vi "MPExxx_Rsrc_example.vi"() -> (0 "Resource String Output":string)   [LabVIEW 2012]
doc: "This VI form creates the resource string for the different communication interfaces."
panel:
  in  "?":T1(tab)
  in  "Comm Port":u8=1 min=1 max=9 step=1
  in  "Address":u8=2 min=1 max=31 step=1
  in  "GPIB Controller":u8
  in  "Port":u16=4000
  in  "TCP/IP Address":string
  # "MAGNA-POWER"
  # "Electronics"
  # "Creates the resource string for ViOpen."
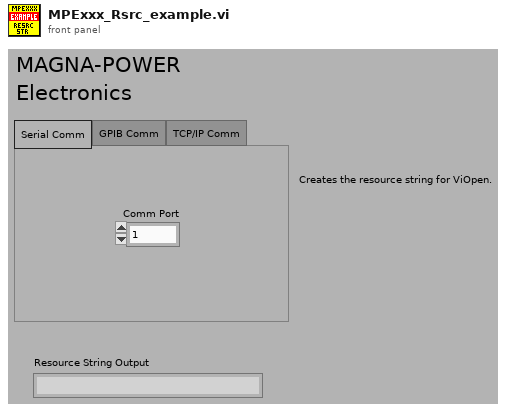
[diagram p1: front panel]
types:
  T1 = enum32{"Serial Comm", "GPIB Comm", "TCP/IP Comm"}
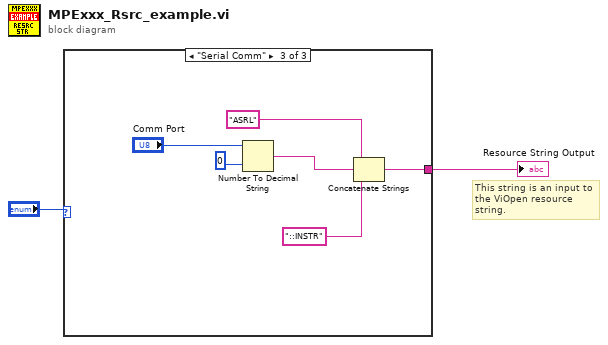
[diagram p0: block diagram]
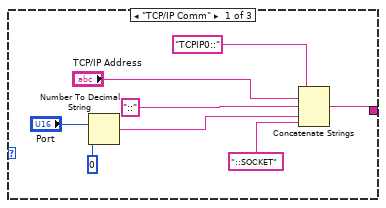
[diagram p2: hidden frame]
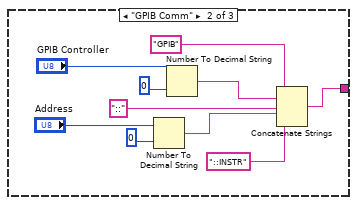
[diagram p3: hidden frame]
diagram:
  # "This string is an input to the ViOpen resource string."
  n1 = case "Case" shown="\"Serial Comm\"" "?" {
    tunnel: [w3 w19 w23] -> w1
    frame "TCP/IP Comm" {
      n2 = Number To Decimal String(number="Port", width (-)=0) -> (decimal integer string=w5:string)
      n3 = Concatenate Strings("TCPIP0::", "TCP/IP Address", "::", w5, "::SOCKET") -> (w3:string)
    }
    frame "GPIB Comm" {
      n4 = Number To Decimal String(number="Address", width (-)=0) -> (decimal integer string=w11:string)
      n5 = Number To Decimal String(number="GPIB Controller", width (-)=0) -> (decimal integer string=w14:string)
      n6 = Concatenate Strings("GPIB", w14, "::", w11, "::INSTR") -> (w19:string)
    }
    frame "Serial Comm" {
      n7 = Number To Decimal String(number="Comm Port", width (-)=0) -> (decimal integer string=w24:string)
      n8 = Concatenate Strings("ASRL", w24, "::INSTR") -> (w23:string)
    }
  }
  "Resource String Output" <- w1
